vi "RPS Turn Score.vi"(11 "RPS Turn In":T1) -> (2 "Score":i32, 3 "RPS Turn":T1)   [LabVIEW 2022 SP3, in "AoC22.lvlib"]
uses:
  AoC22.lvlib
  RPS Turn.ctl
  RPS Play.ctl
  RPS Result.ctl
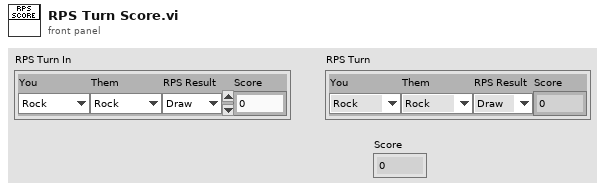
[diagram p1: front panel]
types:
  T1 = typedef "AoC22.lvlib/RPS Turn.ctl" = cluster{"You":T2, "Them":T2, "RPS Result":T3, "Score":i32}
  T2 = typedef "AoC22.lvlib/RPS Play.ctl" = enum16{"Rock", "Paper", "Scissors"}
  T3 = typedef "AoC22.lvlib/RPS Result.ctl" = enum16{"Draw", "Win", "Lose"}
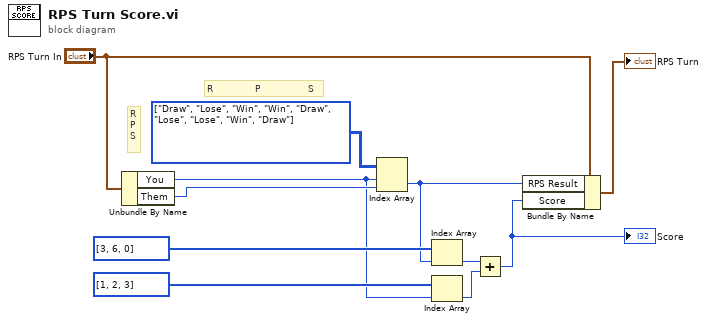
[diagram p0: block diagram]
diagram:
  w9 = T3[][] [[enum."Draw", enum."Lose", enum."Win"], [enum."Win", enum."Draw", enum."Lose"], [enum."Lose", enum."Win", enum."Draw"]] items=["Draw", "Win", "Lose"]
  # "R              P                S"
  # "R\nP\nS"
  n1 = Unbundle By Name("RPS Turn In") -> ("You"=w4:T2, "Them"=w8:T2)
  n2 = Index Array(array=w9, index (row)=w4, index (col)=w8) -> (element=w5:T3)
  n3 = Index Array(array=i32[] [3, 6, 0], index=w5) -> (element=w3:i32)
  n4 = Index Array(array=i32[] [1, 2, 3], index=w4) -> (element=w2:i32)
  n5 = Add(x=w3, y=w2) -> (x+y=w1:i32)
  "Score" <- w1
  n6 = Bundle By Name(cluster="RPS Turn In", "RPS Result"=w5, "Score"=w1) -> (→"RPS Turn":T1)
